vi "VI_CallingVI_InLibrary.vi"(11 "Input String":string) -> (3 "Output String":string)   [LabVIEW 2012]
uses:
  LabVIEW_Library.lvlib
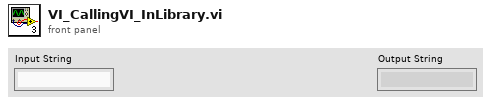
[diagram p1: front panel]
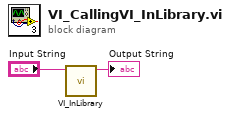
[diagram p0: block diagram]
diagram:
  n1 = call "VI_InLibrary.vi"("Input String"="Input String") -> ("Output String"=→"Output String":string)  [unwired: 10 in]
